vi "Hits_Color_Board.vi"() -> ()   [LabVIEW 2026]
panel:
  out "Attack Board Colors":u32[][](array[colorbox])
  in  "Attack Button":bool
  in  "Player Ship Inputs":T1(array[cluster]) {"Y-Coordinate" min=0 max=7; "X-Coordinate" min=0 max=7}
  in  "stop":bool
  out "Attack Board":dbl[][](array[numeric])
  in  "X (col)":i32
  in  "Y (row)":i32
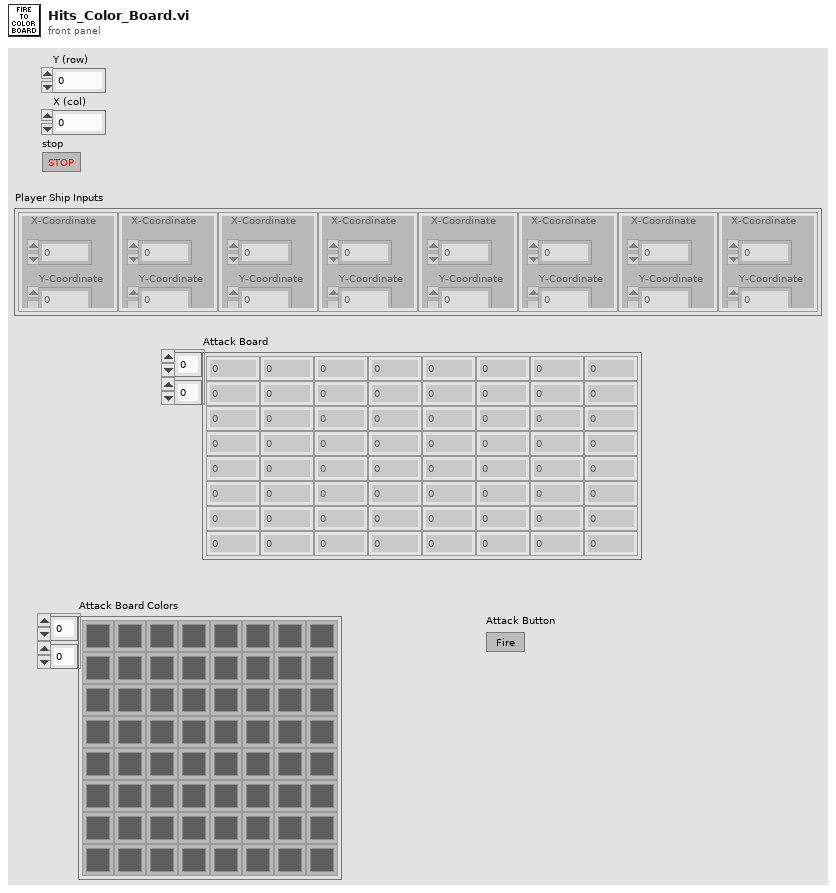
[diagram p1: front panel]
types:
  T1 = cluster{"X-Coordinate":i32, "Y-Coordinate":i32}[]
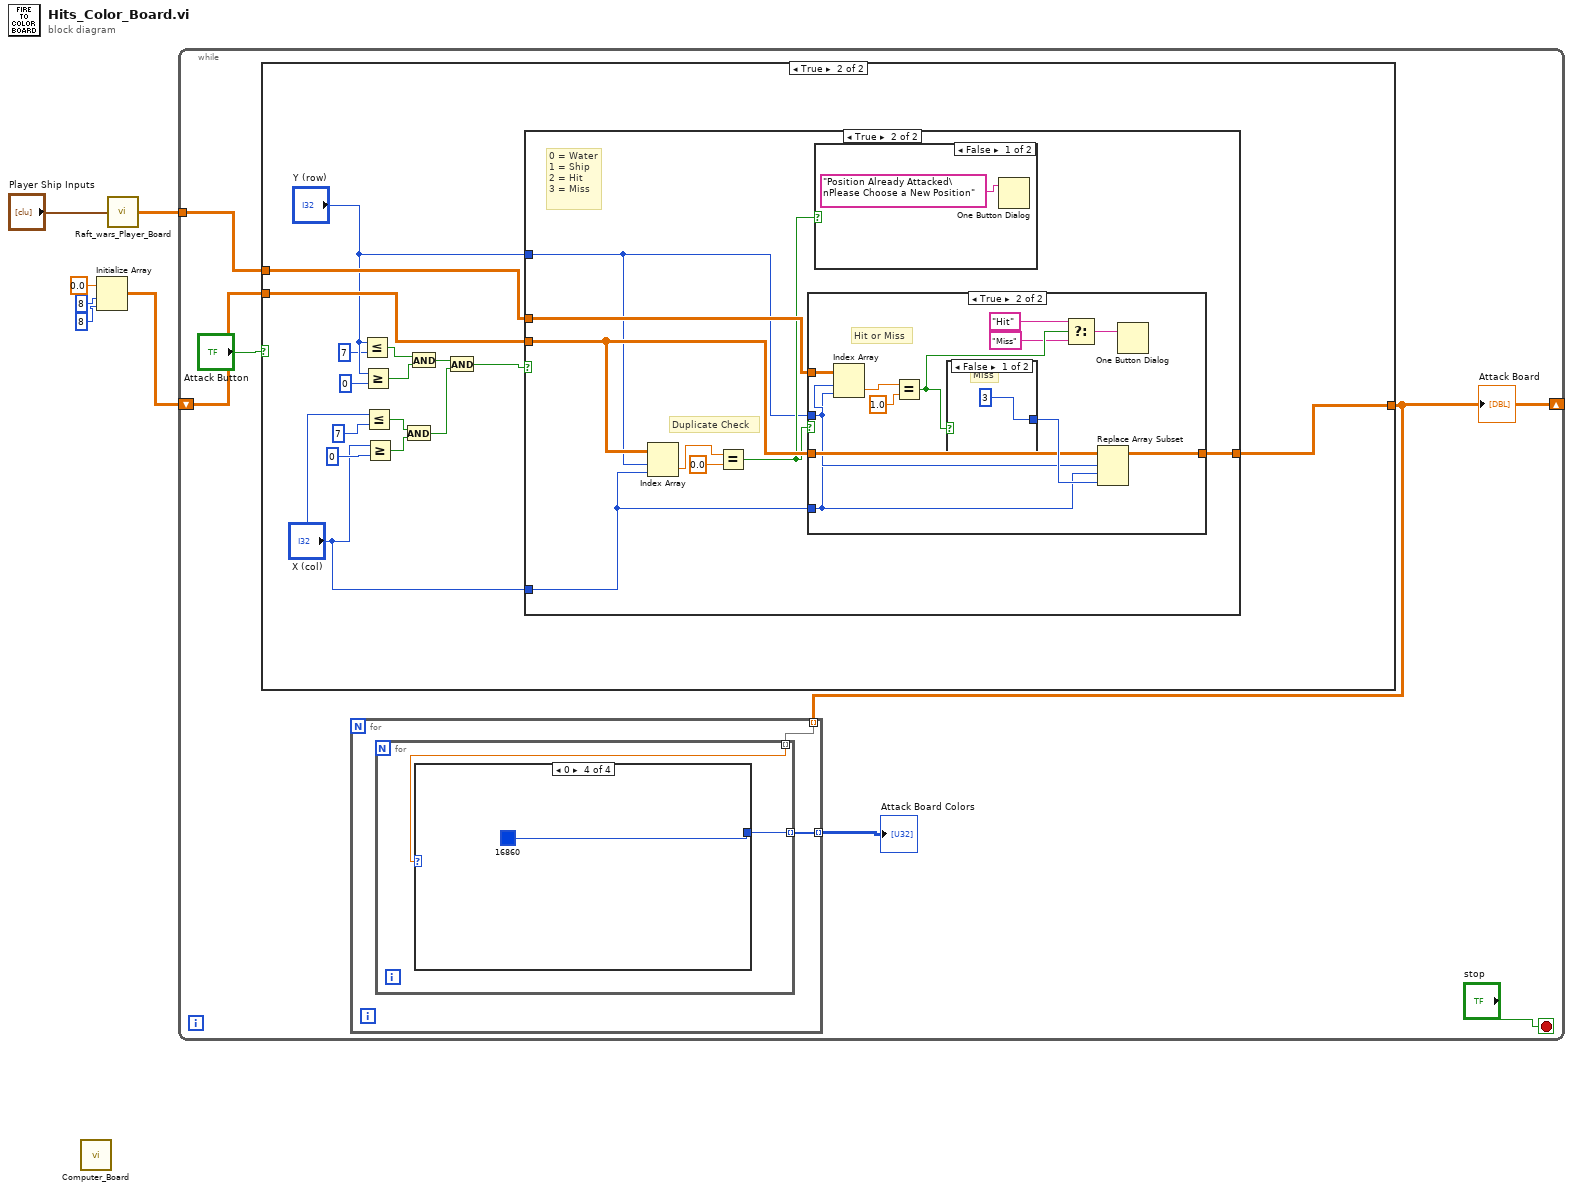
[diagram p0: block diagram]
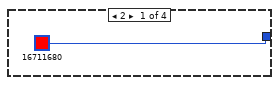
[diagram p2: hidden frame]
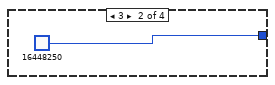
[diagram p3: hidden frame]
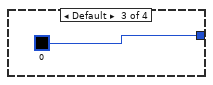
[diagram p4: hidden frame]
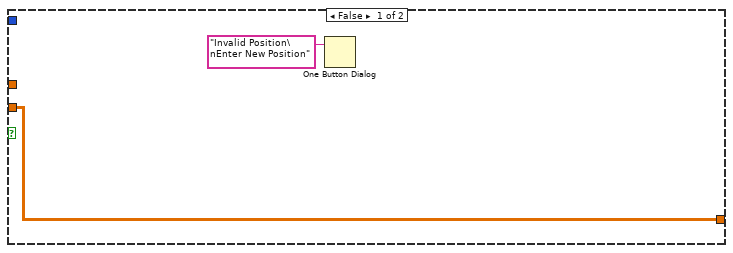
[diagram p6: hidden frame]
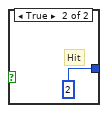
[diagram p9: hidden frame]
diagram:
  n1 = call "Computer_Board.vi"() -> ()  [unwired: 1 out]
  n2 = Initialize Array(0.0 ("element"), 8 ("dimension size"), 8 ("dimension size")) -> (w1:dbl[][])
  n3 = call "Raft_wars_Player_Board.vi"("Player Ship Inputs"="Player Ship Inputs") -> ("Array"=w3:dbl[][])
  n4 = while {
    shift-right: [w8] -> _
    shift-left: w1 -> [w10]
    tunnel: w3 -> [w12]
    stop <- "stop" stop-if-true
    n5 = case shown="True" "Attack Button" {
      tunnel: w12 -> [_ w37]
      tunnel: [w21 w36] -> w8
      tunnel: w10 -> [w21 w35]
      frame False {
      }
      frame True {
        n6 = Less Or Equal?(x="Y (row)", y=7) -> (x <= y?=w29:bool)
        n7 = Greater Or Equal?(x="Y (row)", y=0) -> (x >= y?=w28:bool)
        n8 = Less Or Equal?(x="X (col)", y=7 ("x")) -> (x <= y?=w31:bool)
        n9 = Greater Or Equal?(x="X (col)", y=0 ("x")) -> (x >= y?=w30:bool)
        n10 = And(x=w31, y=w30) -> (x .and. y?=w26:bool)
        n11 = And(x=w29, y=w28) -> (x .and. y?=w27:bool)
        n12 = And(x=w27, y=w26) -> (x .and. y?=w25:bool)
        n13 = case shown="True" w25 {
          tunnel: w37 -> [_ w47]
          tunnel: [w39 w46] -> w36
          tunnel: w35 -> [w39 w45]
          tunnel: "Y (row)" -> [_ w41]
          tunnel: "X (col)" -> [_ w40]
          frame False {
            n14 = One Button Dialog(message="Invalid Position\nEnter New Position") -> ()  [unwired: 1 in, 1 out]
          }
          frame True {
            # "0 = Water\n1 = Ship\n2 = Hit\n3 = Miss"
            # "Duplicate Check"
            n15 = Index Array(array=w45, index (row)=w41, index (col)=w40) -> (element=w44:dbl)
            n16 = Equal?(x=w44, y=0.0) -> (x = y?=w42:bool)
            n17 = case shown="True" w42 {
              tunnel: w47 -> [_ w59]
              tunnel: [w49 w57] -> w46
              tunnel: w45 -> [w49 w56]
              tunnel: w41 -> [_ w55]
              tunnel: w40 -> [_ w54]
              frame False {
              }
              frame True {
                # "Hit or Miss"
                n18 = Index Array(array=w59, index (row)=w55, index (col)=w54) -> (element=w61:dbl)
                n19 = Equal?(x=w61, y=1.0) -> (x = y?=w53:bool)
                n20 = case shown="False" w53 {
                  tunnel: [3 2] -> w58
                  frame False {
                    # "Miss"
                  }
                  frame True {
                    # "Hit"
                  }
                }
                n21 = Select(t="Hit", s=w53, f="Miss") -> (s? t:f=w52:string)
                n22 = Replace Array Subset(array=w56, new element=w58, index (row)=w55, index (col)=w54) -> (w57:dbl[][])
                n23 = One Button Dialog(message=w52) -> ()  [unwired: 1 in, 1 out]
              }
            }
            n24 = case shown="False" w42 {
              frame False {
                n25 = One Button Dialog(message="Position Already Attacked\nPlease Choose a New Position") -> ()  [unwired: 1 in, 1 out]
              }
              frame True {
              }
            }
          }
        }
      }
    }
    "Attack Board" <- w8
    n26 = for {
      tunnel: w8 -> [w14] mode=indexing
      tunnel: [w13] -> w7 mode=indexing
      n27 = for {
        tunnel: w14 -> [w16] mode=indexing
        tunnel: [w15] -> w13 mode=indexing
        n28 = case shown="0" w16 {
          tunnel: [u32 16711680 u32 16448250 u32 0 u32 16860] -> w15
          frame 2 {
          }
          frame 3 {
          }
          frame Default {
          }
          frame 0 {
          }
        }
      }
    }
    "Attack Board Colors" <- w7
  }
